vi "Motor control with position PID.vi"(4 "PID Controls":T2={"PID gains"={"proportional gain (Kc)"=1.0, "integral gain (Kc*Ts/Ti)"=1.66796875, "derivative gain (Kc*Td/Ts)"=0.0}, "reset?"=FALSE, "Velocity Interval (uSec)"=0}, 6 "Motor Connectors":T1={"Enable"="ConnectorB/DIO0", "Input 1"="ConnectorA/DIO1", "Input 2"="ConnectorA/DIO2", "Tach 1"="ConnectorB/DIO8", "Tach 2"="ConnectorB/DIO9"}, 7 "Control":T6={"Motor PWM Control"={"Pulse Lenght DIO3"=10000, "Pulse Period 3"=20000, "Angle"=0}, "stop"=FALSE, "Update Insides Values"=FALSE, "Position Reset"=FALSE}) -> (0 "PID Output":i16, 1 "Speed Output":T4, 2 "Position Output":T3, 3 "Inside values":T5)   [LabVIEW 2013]
uses:
  <vilib>/addons/control/pid/fpga.llb/XNode/niFpgaPID.xnode
  <vilib>/eio/EIONode/EIONode.xnode
  <vilib>/rvi/eio/common/nirviEmuTemplateMethod_errors.vi
panel:
  out "Velocity Interval (uSec)":i32
  out "Velocity (Counts/Interval)":i32
  out "Degree (absolute)":i32
  out "Position Reset":bool
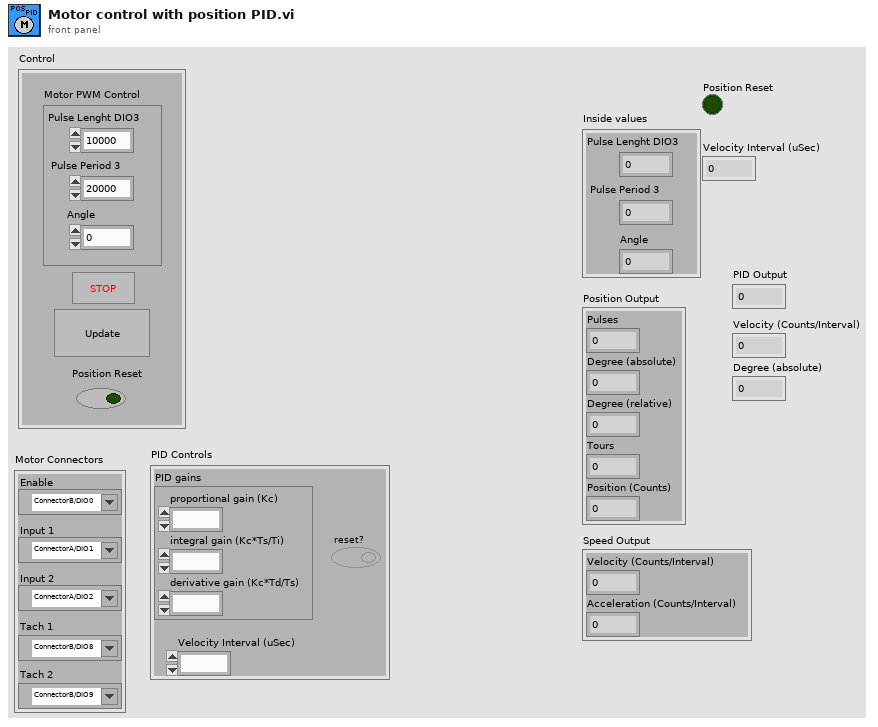
[diagram p1: front panel]
types:
  T1 = cluster{"Enable":refnum<k21>, "Input 1":refnum<k21>, "Input 2":refnum<k21>, "Tach 1":refnum<k21>, "Tach 2":refnum<k21>}
  T2 = cluster{"PID gains":cluster{"proportional gain (Kc)":fxp<+/-,16,8>, "integral gain (Kc*Ts/Ti)":fxp<+/-,16,8>, "derivative gain (Kc*Td/Ts)":fxp<+/-,16,8>}, "reset?":bool, "Velocity Interval (uSec)":i32}
  T3 = cluster{"Pulses":i32, "Degree (absolute)":i32, "Degree (relative)":i32, "Tours":i32, "Position (Counts)":i32}
  T4 = cluster{"Velocity (Counts/Interval)":i32, "Acceleration (Counts/Interval)":i32}
  T5 = cluster{"Pulse Lenght DIO3":i32, "Pulse Period 3":i32, "Angle":i32}
  T6 = cluster{"Motor PWM Control":cluster{"Pulse Lenght DIO3":i32, "Pulse Period 3":i32, "Angle":i32}, "stop":bool, "Update Insides Values":bool, "Position Reset":bool}
  T7 = cluster{"Velocity Interval (uSec)":i32, "I/O Tach 1":bool, "I/O Tach 2":bool, "Position (Counts)":i16, "Boolean Variable 1":bool, "Tick Count(Ticks)":u32, "Position (Counts) 2":i16, "Acceleration (Counts/Interval)":i16, "Velocity (Counts/Interval":i16}
  T8 = cluster{"Tach 1":refnum<k21>, "Tach 2":refnum<k21>}
  T9 = cluster{"proportional gain (Kc)":i16, "integral gain (Kc*Ts/Ti)":i16, "derivative gain (Kc*Td/Ts)":i16}
  T10 = cluster{"proportional gain (Kc)":fxp<+/-,16,8>, "integral gain (Kc*Ts/Ti)":fxp<+/-,16,8>, "derivative gain (Kc*Td/Ts)":fxp<+/-,16,8>}
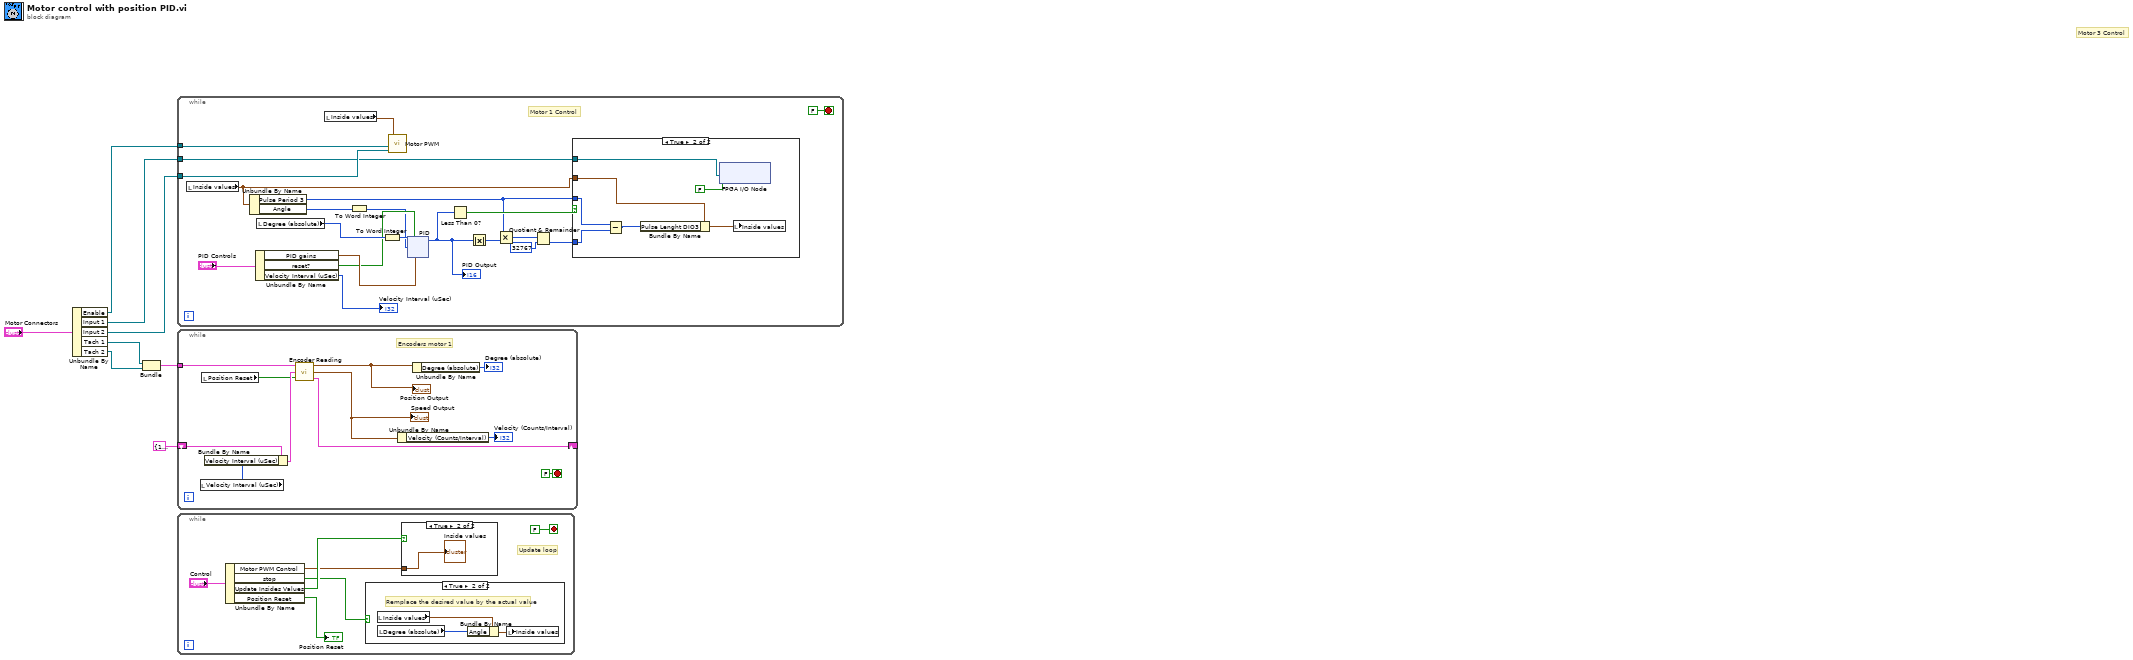
[diagram p0: block diagram]
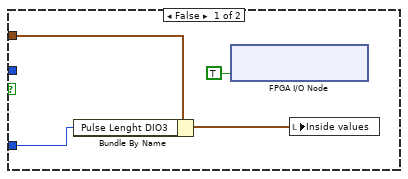
[diagram p2: hidden frame]
diagram:
  # "Motor 3 Control"
  n1 = Unbundle By Name("Motor Connectors") -> ("Enable"=w4:refnum<k21>, "Input 1"=w2:refnum<k21>, "Input 2"=w3:refnum<k21>, "Tach 1"=w7:refnum<k21>, "Tach 2"=w6:refnum<k21>)
  n2 = Bundle("Tach 1"=w7, "Tach 2"=w6) -> (w5:T8)  [unwired: 1 in]
  n3 = while {
    tunnel: w4 -> [w17]
    tunnel: w3 -> [w16]
    tunnel: w2 -> [w15]
    stop <- FALSE stop-if-true
    # "Motor 1 Control"
    n4 = local read "Inside values"() -> (w20:T5)
    n5 = Unbundle By Name(w20) -> ("Pulse Period 3"=w19:i32, "Angle"=w11:i32)
    n6 = Unbundle By Name("PID Controls") -> ("PID gains"=w13:T10, "reset?"=w12:bool, "Velocity Interval (uSec)"=→"Velocity Interval (uSec)":i32)
    n7 = local read "Degree (absolute)"() -> (w26:i32)
    n8 = local read "Inside values"() -> (w18:T5)
    n9 = To Word Integer(number=w11) -> (16bit integer=w10:i16)
    n10 = To Word Integer(number=w26) -> (16bit integer=w29:i16)
    n11 = call "Motor PWM.vi"("Motor Input 2"=w16, "Motor Enable"=w17, "Inside values"=w18) -> ()  [unwired: 1 in]
    n12 = xnode "PID"("process variable"=w29, "reset?"=w12, "setpoint"=w10, "PID gains"=w13) -> ("output"=w22:i16)  [unwired: 1 in]
    "PID Output" <- w22
    n13 = Less Than 0?(x=w22) -> (x < 0?=w28:bool)
    n14 = Absolute Value(x=w22) -> (abs(x)=w24:i16)
    n15 = Multiply(x=w19, y=w24) -> (x*y=w23:i32)
    n16 = Quotient & Remainder(x=w23, y=i16 32767) -> (floor(x/y)=w21:i32)  [unwired: 1 out]
    n17 = case shown="True" w28 {
      tunnel: w21 -> [w31 w39]
      tunnel: w20 -> [w30 w36]
      tunnel: w19 -> [_ w40]
      tunnel: w15 -> [_ w34]
      frame False {
        n18 = Bundle By Name(cluster=w30, "Pulse Lenght DIO3"=w31) -> (w32:T5)
        n19 = xnode "FPGA I/O Node"("ConnectorB/DIO1"=TRUE ("ConnectorC/DIO7")) -> ()  [unwired: 1 in, 1 out]
        n20 = local write "Inside values"(w32) -> ()
      }
      frame True {
        n21 = Subtract(x=w40, y=w39) -> (x-y=w37:i32)
        n22 = Bundle By Name(cluster=w36, "Pulse Lenght DIO3"=w37) -> (w38:T5)
        n23 = xnode "FPGA I/O Node"("I/O Item"=FALSE ("ConnectorC/DIO7"), "FPGA I/O In"=w34) -> ()  [unwired: 1 out]
        n24 = local write "Inside values"(w38) -> ()
      }
    }
  }
  n25 = while {
    shift-right: [w77] -> _
    shift-left: T7 {"Velocity Interval (uSec)"=1000000, "I/O Tach 1"=FALSE, "I/O Tach 2"=FALSE, "Position (Counts)"=0, "Boolean Variable 1"=FALSE, "Tick Count(Ticks)"=0, "Position (Counts) 2"=0, "Acceleration (Counts/Interval)"=0, "Velocity (Counts/Interval"=0} ("Values") -> [w72]
    tunnel: w5 -> [w78]
    stop <- FALSE stop-if-true
    # "Encoders motor 1"
    n26 = local read "Velocity Interval (uSec)"() -> (w69:i32)
    n27 = local read "Position Reset"() -> (w70:bool)
    n28 = Bundle By Name(cluster=w72, "Velocity Interval (uSec)"=w69) -> (w71:T7)
    n29 = call "Encoder Reading.vi"("Position Reset"=w70, "Values"=w71, "Encoder Intputs"=w78) -> ("output cluster"=w77:T7, "Speed Output"=w73:T4, "Position Output"=w74:T3)
    "Position Output" <- w74
    "Speed Output" <- w73
    n30 = Unbundle By Name(w73) -> ("Velocity (Counts/Interval)"=→"Velocity (Counts/Interval)":i32)
    n31 = Unbundle By Name(w74) -> ("Degree (absolute)"=→"Degree (absolute)":i32)
  }
  n32 = while {
    stop <- FALSE stop-if-true
    # "Update loop"
    n33 = Unbundle By Name("Control") -> ("Motor PWM Control"=w81:T5, "stop"=w82:bool, "Update Insides Values"=w83:bool, "Position Reset"=→"Position Reset":bool)
    n34 = case shown="True" w82 {
      frame False {
      }
      frame True {
        # "Remplace the desired value by the actual value"
        n35 = local read "Inside values"() -> (w88:T5)
        n36 = local read "Degree (absolute)"() -> (w87:i32)
        n37 = Bundle By Name(cluster=w88, "Angle"=w87) -> (w86:T5)
        n38 = local write "Inside values"(w86) -> ()
      }
    }
    n39 = case shown="True" w83 {
      tunnel: w81 -> [_ w89]
      frame False {
      }
      frame True {
        "Inside values" <- w89
      }
    }
  }
